vi "滤波模块.vi"(8 "通量名称":string[](array[string]), 9 "执行:调用时显示前面板":bool, 10 "P2信号":dbl[](array[numeric]), 11 "通量in":dbl[](array[numeric])) -> (0 "面板开":bool, 1 "滤波开":bool, 3 "通量out":dbl[](array[numeric]))   [LabVIEW 2020]
uses:
  <vilib>/Analysis/3filter.llb/Savitzky-Golay Filter (DBL).vi
  <vilib>/Analysis/3filter.llb/FIR Filter (DBL).vi
  <vilib>/Analysis/NI_AALBase.lvlib
panel:
  in  "滤波数组":dbl[][](array[numeric])
  in  "上一点":dbl[](array[numeric])
  in  "滤波显示选择":u16(ring) items=["电流1a", "电流2a"]
  out "滤波效果图":dbl[](graph)
  in  "滤波方法选择":T1(tab)=enum."中值滤波"
  in  "滤波系数(0-0.99)":dbl=0.5 min=0.0 max=0.99 step=0.01 format="%#.2f"
  in  "左秩":i32
  in  "side points":i32=24 caption="单侧数据点数"
  in  "polynomial":i32=3 caption="多项式阶数"
  in  "滤波系数":dbl=0.1
  in  "滤波点数":i32=10
  in  "滤波有效":bool
  # "0相位滤波"
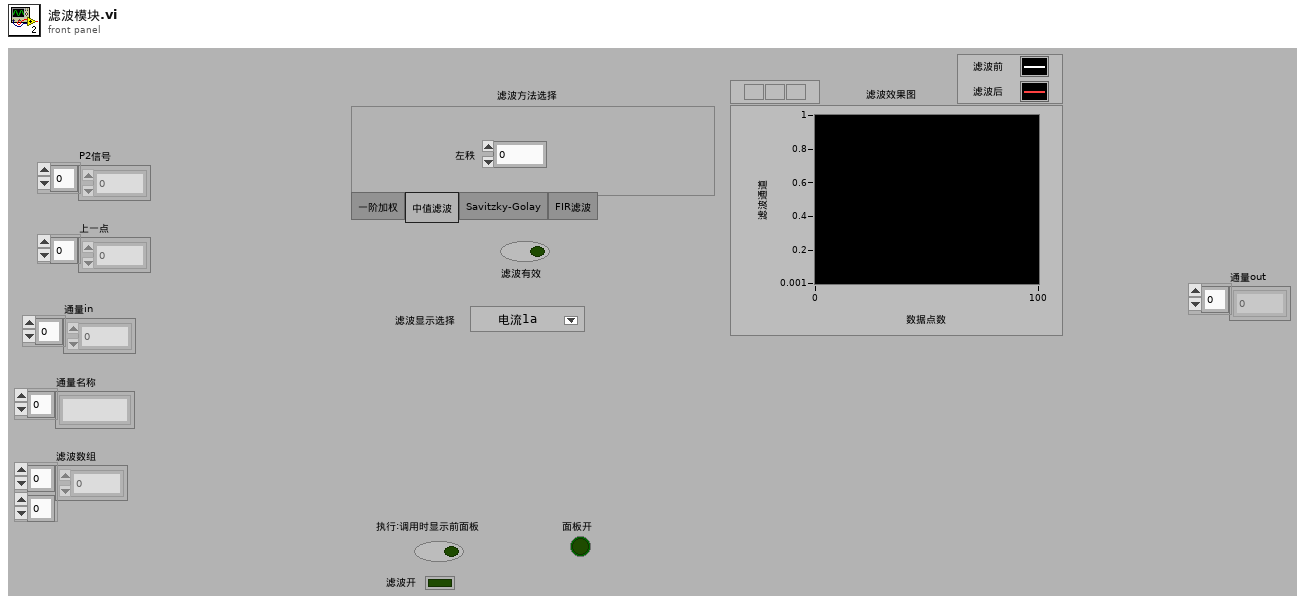
[diagram p1: front panel]
types:
  T1 = enum32{"一阶加权", "中值滤波", "Savitzky-Golay", "FIR滤波"}
  T2 = enum8{"Enabled", "Disabled", "Disabled and Grayed Out"}
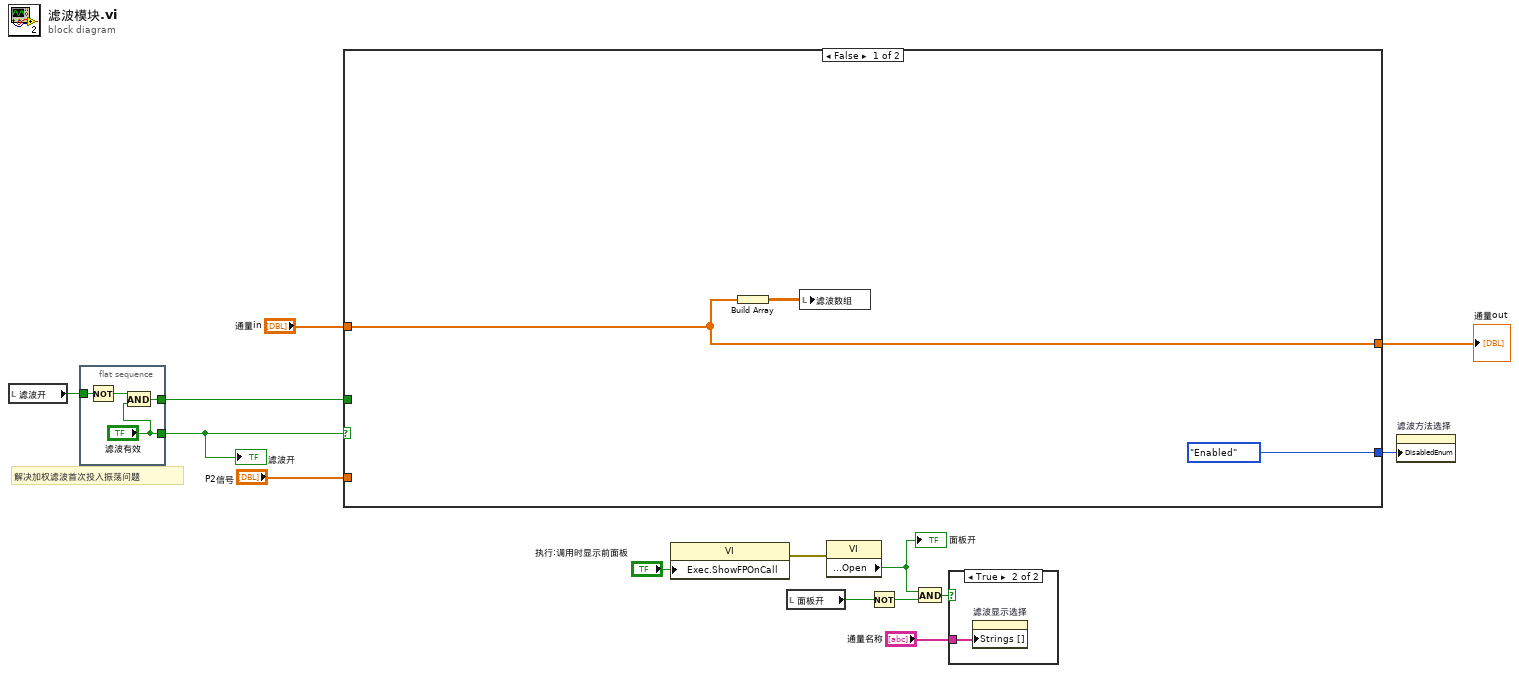
[diagram p0: block diagram]
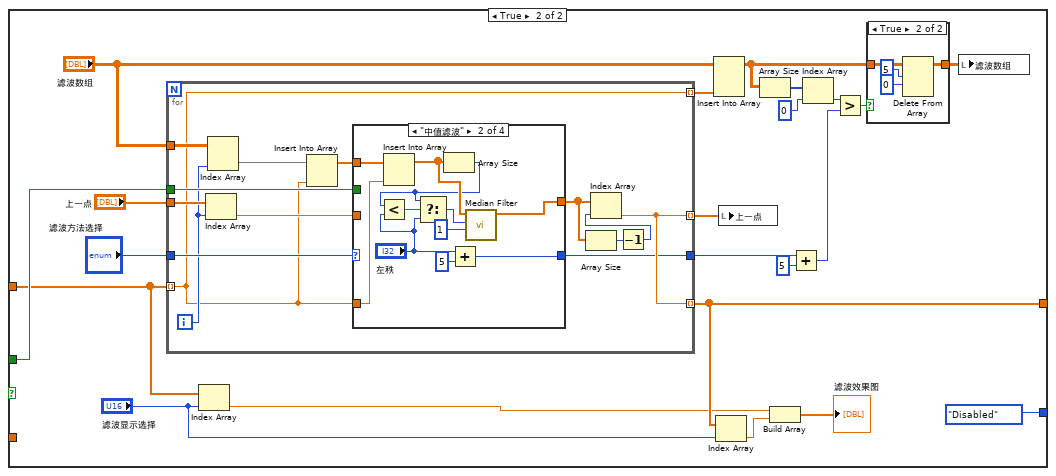
[diagram p2: hidden frame]
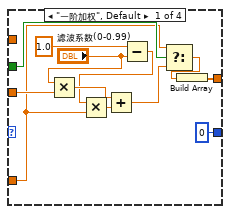
[diagram p4: hidden frame]
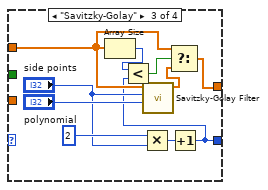
[diagram p5: hidden frame]
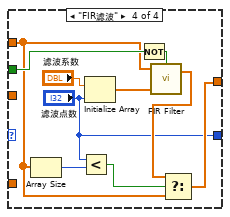
[diagram p6: hidden frame]
diagram:
  # "解决加权滤波首次投入振荡问题"
  n1 = local read "滤波开"() -> (w5:bool)
  n2 = flat-sequence {
    tunnel: ["滤波有效"] -> w7
    tunnel: [w16] -> w6
    tunnel: w5 -> [w15]
    frame #0 {
      n3 = Not(x=w15) -> (.not. x?=w18:bool)
      n4 = And(x=w18, y="滤波有效") -> (x .and. y?=w16:bool)
    }
  }
  n5 = case shown="False" w7 {
    tunnel: "通量in" -> [w19 w41]
    tunnel: [w19 w40] -> w1
    tunnel: w6 -> [_ w42]
    tunnel: "P2信号" -> [_ _]
    tunnel: [T2."Enabled" ("禁用") T2."Disabled" ("禁用")] -> w3
    frame False {
      n6 = Build Array(w19) -> (w20:dbl[][])
      n7 = local write "滤波数组"(w20) -> ()
    }
    frame True {
      n8 = for {
        tunnel: "滤波方法选择" -> [w62]
        tunnel: w42 -> [w61]
        tunnel: w41 -> [w53] mode=indexing
        tunnel: [w58] -> w40 mode=indexing
        tunnel: [w58] -> w29 mode=indexing
        tunnel: "上一点" -> [w60]
        tunnel: [w53] -> w28 mode=indexing
        tunnel: "滤波数组" -> [w57]
        tunnel: [w54] -> w26
        i -> [w56]
        n9 = Index Array(array=w60, index=w56) -> (element=w59:dbl)
        n10 = Index Array(array=w57, index (col)=w56) -> (element=w55:dbl[])  [unwired: 1 in]
        n11 = Insert Into Array(array=w55, new element=w53) -> (w49:dbl[])  [unwired: 1 in]
        n12 = case shown="\"中值滤波\"" w62 {
          tunnel: w53 -> [w63 w84 _ _]
          tunnel: w61 -> [w66 _ _ w103]
          tunnel: w59 -> [w69 _ _ _]
          tunnel: w49 -> [_ w85 w90 w100]
          tunnel: [w68 w78 w92 w101] -> w50
          tunnel: [0 w76 w86 "滤波点数"] -> w54
          frame "一阶加权", Default {
            n13 = Multiply(x="滤波系数(0-0.99)", y=w69) -> (x*y=w72:dbl)
            n14 = Subtract(x=1.0 ("新点权重%"), y="滤波系数(0-0.99)") -> (x-y=w70:dbl)
            n15 = Multiply(x=w70, y=w63) -> (x*y=w73:dbl)
            n16 = Add(x=w72, y=w73) -> (x+y=w64:dbl)
            n17 = Select(t=w63, s=w66, f=w64) -> (s? t:f=w65:dbl)
            n18 = Build Array(w65) -> (w68:dbl[])
          }
          frame "中值滤波" {
            n19 = Insert Into Array(array=w85, new element=w84) -> (w83:dbl[])  [unwired: 1 in]
            n20 = Array Size(array=w83) -> (size(s)=w79:i32)
            n21 = Less?(x=w79, y="左秩") -> (x < y?=w82:bool)
            n22 = Select(t=w79, s=w82, f="左秩") -> (s? t:f=w80:i32)
            n23 = Add(x="左秩", y=5) -> (x+y=w76:i32)
            n24 = call <vilib>:"Median Filter.vi"("right rank"=1, "left rank"=w80, "X"=w83) -> ("Filtered X"=w78:dbl[])  [unwired: 7 in, 1 out]
          }
          frame "Savitzky-Golay" {
            n25 = Array Size(array=w90) -> (size(s)=w89:i32)
            n26 = Multiply(x=2, y="side points") -> (x*y=w93:i32)
            n27 = call-poly <vilib>:"Savitzky-Golay Filter.vi"("polynomial order"="polynomial", "side points"="side points", "X"=w90) -> ("Filtered X"=w91:dbl[])  [unwired: 7 in, 1 out]
            n28 = Increment(x=w93) -> (x+1=w86:i32)
            n29 = Less?(x=w89, y=w86) -> (x < y?=w87:bool)
            n30 = Select(t=w90, s=w87, f=w91) -> (s? t:f=w92:dbl[])
          }
          frame "FIR滤波" {
            n31 = Array Size(array=w100) -> (size(s)=w97:i32)
            n32 = Less?(x="滤波点数", y=w97) -> (x < y?=w99:bool)
            n33 = Initialize Array("滤波系数", "滤波点数") -> (w104:dbl[])
            n34 = Not(x=w103) -> (.not. x?=w96:bool)
            n35 = call-poly <vilib>:"FIR Filter.vi"("init/cont (init:F)"=w96, "FIR Coefficients"=w104, "X"=w100) -> ("Filtered X"=w102:dbl[])  [unwired: 1 in, 1 out]
            n36 = Select(t=w102, s=w99, f=w100) -> (s? t:f=w101:dbl[])
          }
        }
        n37 = Array Size(array=w50) -> (size(s)=w52:i32)
        n38 = Decrement(x=w52) -> (x-1=w51:i32)
        n39 = Index Array(array=w50, index=w51) -> (element=w58:dbl)
      }
      n40 = Index Array(array=w41, index="滤波显示选择") -> (element=w38:dbl)
      n41 = Insert Into Array(array="滤波数组", new element=w28) -> (w33:dbl[][])  [unwired: 2 in]
      n42 = Index Array(array=w40, index="滤波显示选择") -> (element=w37:dbl)
      n43 = local write "上一点"(w29) -> ()
      n44 = Array Size(array=w33) -> (size(s)=w36:i32[])
      n45 = Build Array(w38, w37) -> (→"滤波效果图":dbl[])
      n46 = Add(x=w26, y=5) -> (x+y=w24:i32)
      n47 = Index Array(array=w36, index=0 ("索引")) -> (element=w34:i32)
      n48 = Greater?(x=w34, y=w24) -> (0:w32:bool)
      n49 = case shown="True" w32 {
        tunnel: w33 -> [w44 w48]
        tunnel: [w44 w45] -> w31
        frame False {
        }
        frame True {
          n50 = Delete From Array(array=w48, length=5 ("长度"), index (row)=0 ("索引 (行)")) -> (array with subset deleted=w45:dbl[][])  [unwired: 1 in, 1 out]
        }
      }
      n51 = local write "滤波数组"(w31) -> ()
    }
  }
  "通量out" <- w1
  n52 = property class="VI"("Exec.ShowFPOnCall"="执行:调用时显示前面板") -> (error out=w13:errorcluster)  [unwired: 2 in, 1 out]
  n53 = local read "面板开"() -> (w12:bool)
  n54 = property class="VI"(error in=w13) -> ("Front Panel.Open"=w10:bool)  [unwired: 1 in, 2 out]
  "面板开" <- w10
  n55 = Not(x=w12) -> (.not. x?=w11:bool)
  n56 = And(x=w10, y=w11) -> (x .and. y?=w9:bool)
  n57 = case shown="True" w9 {
    tunnel: "通量名称" -> [_ w106]
    frame False {
    }
    frame True {
      n58 = property on="滤波显示选择" class="Ring (strict)"("Strings []"=w106) -> ()  [unwired: 2 in, 2 out]
    }
  }
  n59 = property on="滤波方法选择" class="TabCtl (strict)"("DisabledEnum"=w3) -> ()  [unwired: 2 in, 2 out]
  "滤波开" <- w7
